vi "YokoGS200 Set FuncAndRg.vi"(8 "error in (no error)":errorcluster, 9 "Source Range":T1(ring), 10 "Source Function":enum16{"Current", "Voltage"}(ring), 11 "VISA Rsrc":refnum<visa-resource-name>="SR530") -> (0 "error out":errorcluster, 3 "VISA Rsrc Out":refnum<visa-resource-name>="GPIB0::12::INSTR", 4 "ChaineCom":string caption="Chaîne de commande")   [LabVIEW 2019]
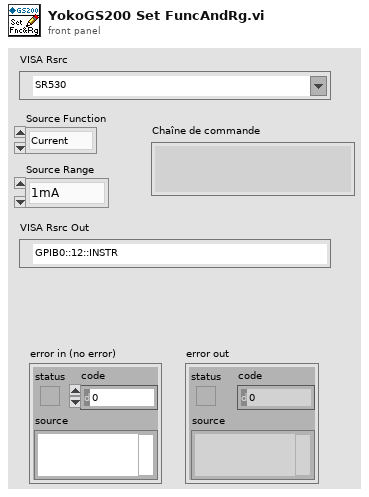
[diagram p1: front panel]
types:
  T1 = enum16{"1mA", "10mA", "100mA", "200mA", "10mV", "100mV", "1V", "10V", "30V", "Minimum", "Maximum"}
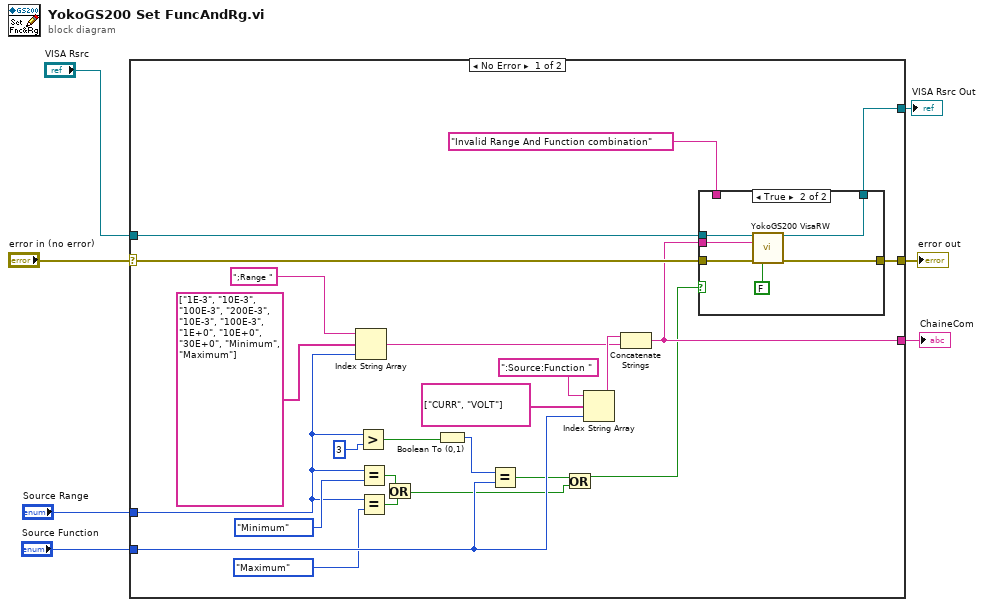
[diagram p0: block diagram]
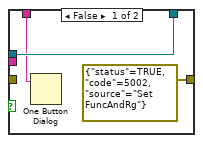
[diagram p2: hidden frame]
diagram:
  n1 = case shown="No Error" "error in (no error)" {
    selector: "error in (no error)" -> [w30 w41]
    tunnel: "VISA Rsrc" -> [w31 w42]
    tunnel: [w19 w41] -> w5
    tunnel: [w29 w42] -> w4
    tunnel: [w18 _] -> w3
    tunnel: "Source Range" -> [w13 _]
    tunnel: "Source Function" -> [w22 _]
    frame No Error {
      n2 = Index String Array(1:w13, 2:string[] ["1E-3", "10E-3", "100E-3", "200E-3", "10E-3", "100E-3", "1E+0", "10E+0", "30E+0", "Minimum", "Maximum"] ("output array"), 3:";Range " ("ChaineCom")) -> (0:w20:string)
      n3 = Greater?(x=w13, y=3) -> (0:w10:bool)
      n4 = Equal?(x=w13, y=T1."Minimum") -> (x = y?=w12:bool)
      n5 = Equal?(x=w13, y=T1."Maximum") -> (x = y?=w11:bool)
      n6 = Or(x=w12, y=w11) -> (x .or. y?=w8:bool)
      n7 = Boolean To (0,1)(Boolean=w10) -> (0, 1=w23:i16)
      n8 = Equal?(x=w23, y=w22) -> (x = y?=w17:bool)
      n9 = Or(x=w17, y=w8) -> (x .or. y?=w9:bool)
      n10 = Index String Array(1:w22, 2:string[] ["CURR", "VOLT"] ("string array"), 3:":Source:Function " ("string (\"\")")) -> (0:w21:string)
      n11 = Concatenate Strings(w21, w20) -> (w18:string)
      n12 = case shown="True" w9 {
        tunnel: w31 -> [w34 w40]
        tunnel: w30 -> [_ w39]
        tunnel: [w34 w38] -> w29
        tunnel: [errorcluster {"status"=TRUE, "code"=5002, "source"="Set FuncAndRg"} ("error out") w36] -> w19
        tunnel: w18 -> [_ w35]
        tunnel: "Invalid Range And Function combination" ("message") -> [w32 _]
        frame False {
          n13 = One Button Dialog(message=w32) -> ()  [unwired: 1 in, 1 out]
        }
        frame True {
          n14 = call <userlib>:"YokoGS200 VisaRW.vi"("VISA Rsrc"=w40, "ChaineCom"=w35, "error in (no error)"=w39, "Lecture?(T)"=FALSE) -> ("VISA Rsrc Out"=w38:refnum<visa-resource-name>, "error out"=w36:errorcluster)  [unwired: 7 in, 3 out]
        }
      }
    }
    frame Error {
    }
  }
  "error out" <- w5
  "VISA Rsrc Out" <- w4
  "ChaineCom" <- w3
